vi "formatMotorInputToMega.vi"(0 "zone 3 co2":dbl, 1 "Light in":i32, 2 "zone 3 return":dbl, 3 "Light 3":i32, 4 "zone 2 co2":dbl, 5 "fresh air":dbl, 6 "zone 1 co2":dbl, 7 "error in (no error)":errorcluster, 8 "Light 1":i32, 9 "zone 3 inlet":dbl, 10 "zone 2 return":dbl, 11 "Fans":i32, 12 "zone 2 inlet":dbl, 14 "zone 1 return":dbl, 16 "zone 1 inlet":dbl) -> (18 "String":string, 27 "error out":errorcluster)   [LabVIEW 2019]
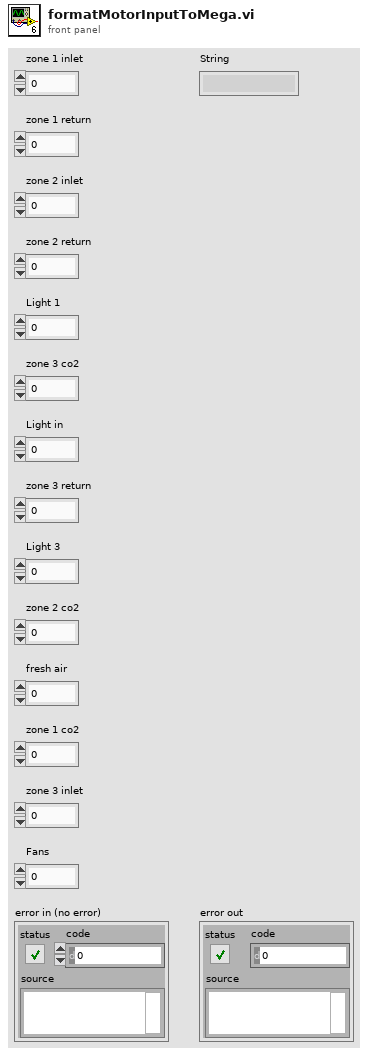
[diagram p1: front panel]
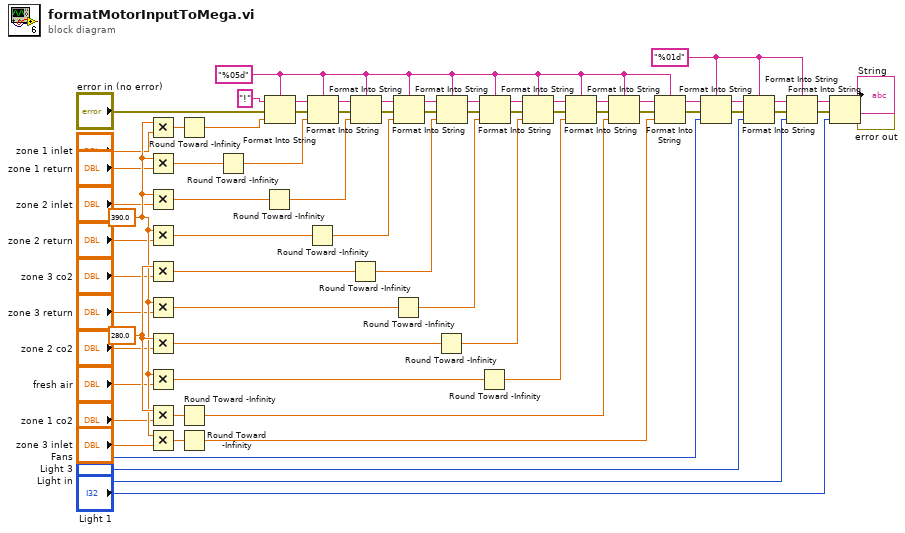
[diagram p0: block diagram]
diagram:
  w67 = 280.0 ("x")
  w46 = 390.0 ("y")
  w27 = "%01d" ("format string")
  w20 = "%05d" ("format string")
  n1 = Multiply(x=w46, y="zone 1 inlet") -> (x*y=w66:dbl)
  n2 = Multiply(x=w46, y="zone 1 return") -> (x*y=w65:dbl)
  n3 = Multiply(x=w46, y="zone 2 inlet") -> (x*y=w64:dbl)
  n4 = Multiply(x=w46, y="zone 2 return") -> (x*y=w63:dbl)
  n5 = Multiply(x=w67, y="zone 3 co2") -> (x*y=w62:dbl)
  n6 = Multiply(x=w46, y="zone 3 return") -> (x*y=w61:dbl)
  n7 = Multiply(x=w67, y="zone 2 co2") -> (x*y=w60:dbl)
  n8 = Multiply(x=w46, y="fresh air") -> (x*y=w59:dbl)
  n9 = Multiply(x=w67, y="zone 1 co2") -> (x*y=w58:dbl)
  n10 = Multiply(x=w46, y="zone 3 inlet") -> (x*y=w57:dbl)
  n11 = Round Toward -Infinity(1:w66) -> (0:w47:dbl)
  n12 = Round Toward -Infinity(1:w58) -> (0:w55:dbl)
  n13 = Round Toward -Infinity(1:w57) -> (0:w56:dbl)
  n14 = Round Toward -Infinity(1:w65) -> (0:w48:dbl)
  n15 = Round Toward -Infinity(1:w64) -> (0:w49:dbl)
  n16 = Format Into String(format string=w20, initial string="!" ("write buffer"), error in="error in (no error)", w47) -> (resulting string=w2:string, error out=w1:errorcluster)
  n17 = Round Toward -Infinity(1:w63) -> (0:w50:dbl)
  n18 = Format Into String(format string=w20, initial string=w2, error in=w1, w48) -> (resulting string=w4:string, error out=w3:errorcluster)
  n19 = Round Toward -Infinity(1:w62) -> (0:w51:dbl)
  n20 = Format Into String(format string=w20, initial string=w4, error in=w3, w49) -> (resulting string=w6:string, error out=w5:errorcluster)
  n21 = Round Toward -Infinity(1:w61) -> (0:w52:dbl)
  n22 = Format Into String(format string=w20, initial string=w6, error in=w5, w50) -> (resulting string=w8:string, error out=w7:errorcluster)
  n23 = Round Toward -Infinity(1:w60) -> (0:w53:dbl)
  n24 = Format Into String(format string=w20, initial string=w8, error in=w7, w51) -> (resulting string=w10:string, error out=w9:errorcluster)
  n25 = Round Toward -Infinity(1:w59) -> (0:w54:dbl)
  n26 = Format Into String(format string=w20, initial string=w10, error in=w9, w52) -> (resulting string=w12:string, error out=w11:errorcluster)
  n27 = Format Into String(format string=w20, initial string=w12, error in=w11, w53) -> (resulting string=w13:string, error out=w14:errorcluster)
  n28 = Format Into String(format string=w20, initial string=w13, error in=w14, w54) -> (resulting string=w18:string, error out=w16:errorcluster)
  n29 = Format Into String(format string=w20, initial string=w18, error in=w16, w55) -> (resulting string=w19:string, error out=w17:errorcluster)
  n30 = Format Into String(format string=w20, initial string=w19, error in=w17, w56) -> (resulting string=w24:string, error out=w21:errorcluster)
  n31 = Format Into String(format string=w27, initial string=w24, error in=w21, "Fans") -> (resulting string=w25:string, error out=w22:errorcluster)
  n32 = Format Into String(format string=w27, initial string=w25, error in=w22, "Light 3") -> (resulting string=w26:string, error out=w23:errorcluster)
  n33 = Format Into String(format string=w27, initial string=w26, error in=w23, "Light in") -> (resulting string=w29:string, error out=w28:errorcluster)
  n34 = Format Into String(initial string=w29, error in=w28, "Light 1") -> (resulting string=→"String":string, error out=→"error out":errorcluster)  [unwired: 1 in]
